vi "Is Initialized.vi"(8 "error in":errorcluster, 11 "SimpleCsvDataLogger in":refnum<class "SimpleCsvDataLogger.lvclass">) -> (0 "error out":errorcluster, 2 "Is Initialized?":bool, 3 "SimpleCsvDataLogger out":refnum<class "SimpleCsvDataLogger.lvclass">)   [LabVIEW 2019, in "SimpleCsvDataLogger.lvclass"]
uses:
  SimpleCsvDataLogger.lvclass
  SimpleCsvDataLogger.lvclass/SimpleCsvDataLogger.ctl
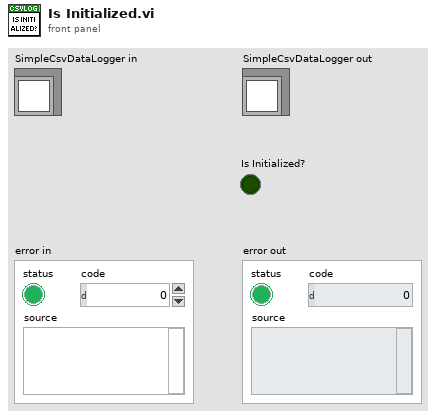
[diagram p1: front panel]
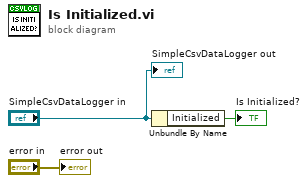
[diagram p0: block diagram]
diagram:
  n1 = Unbundle By Name("SimpleCsvDataLogger in") -> ("Initialized"=→"Is Initialized?":bool)
  "SimpleCsvDataLogger out" <- "SimpleCsvDataLogger in"
  "error out" <- "error in"
